vi "Actor Core.vi"(8 "error in":errorcluster, 11 "Elevator Controller in":refnum<class "Sim Display Console Actor.lvclass">) -> (0 "error out":errorcluster, 3 "Actor out":refnum<class "Actor.lvclass">)   [LabVIEW 2019, in "Sim Display Console Actor.lvlib" / "Sim Display Console Actor.lvclass"]
doc: "(<B>Filename</B>: Actor Framework.lvlib:Actor.lvclass:Actor Core.vi)\n\nReceives messages to the actor, reacts to them, and initiates any error handling that may shut the actor down.\n\nDescendant classes may override this VI to append parallel tasks for the actor to complete while it handles messages. Overrides use the Call Parent Method node."
uses:
  Sim Display Console Actor.lvclass
  <vilib>/ActorFramework/Actor/Actor.lvclass
  <vilib>/ActorFramework/Stop Msg/Stop Msg.lvclass
  Display Console Actor/Display Console Actor/Display Console Actor.lvclass
  C:/Workspace/CLA/Elevator AF 3rd/Display Console Actor/Display Console Actor/Display Console Actor.lvclass
  C:/Program Files (x86)/National Instruments/LabVIEW 2019/vi.lib/ActorFramework/Actor/Actor.lvclass
  Elevator Controller/Elevator Controller Messages/Get Elevator Location Msg/Get Elevator Location Msg.lvclass
  Elevator Controller/Elevator Controller Messages/Set Elevator Position Msg/Set Elevator Position Msg.lvclass
  Floors -Enum.ctl
  Elevator Direction.ctl
panel:
  out "Door Open":bool
  out "Emergency":bool
  out "Elevator Direction":T1
  out "Elevator Location":T2
  out "Timing":dbl
  # "[Covers: UI3]"
  # "[Covers: UI3C]"
  # "[Covers: UI3A] \n[Covers: UI3A1] \n[Covers: UI3A2]"
  # "[Covers: UI3D] \n[Covers: UI3D1]"
  # "[Covers: UI3B]"
  # "[Covers: UI3E]"
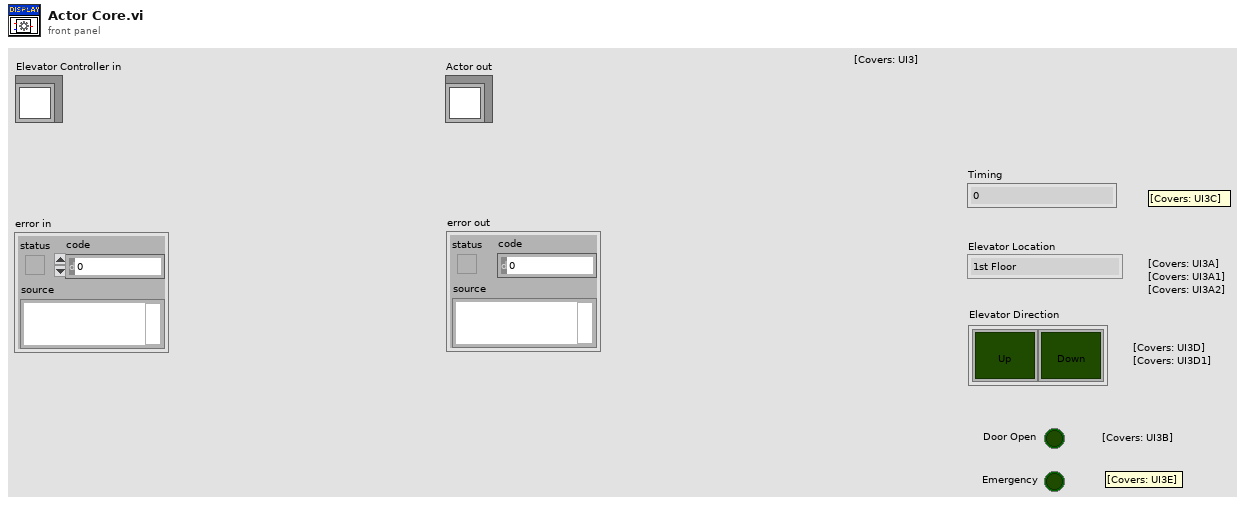
[diagram p1: front panel]
types:
  T1 = typedef "Sim Display Console Actor.lvlib/Sim Display Console Actor.lvclass/Elevator Direction.ctl" = cluster{"Open Door":bool, "Close Door":bool}
  T2 = typedef "Sim Display Console Actor.lvlib/Sim Display Console Actor.lvclass/Floors -Enum.ctl" = enum16{"1st Floor", "2nd Floor", "3rd Floor", "4th Floor"}
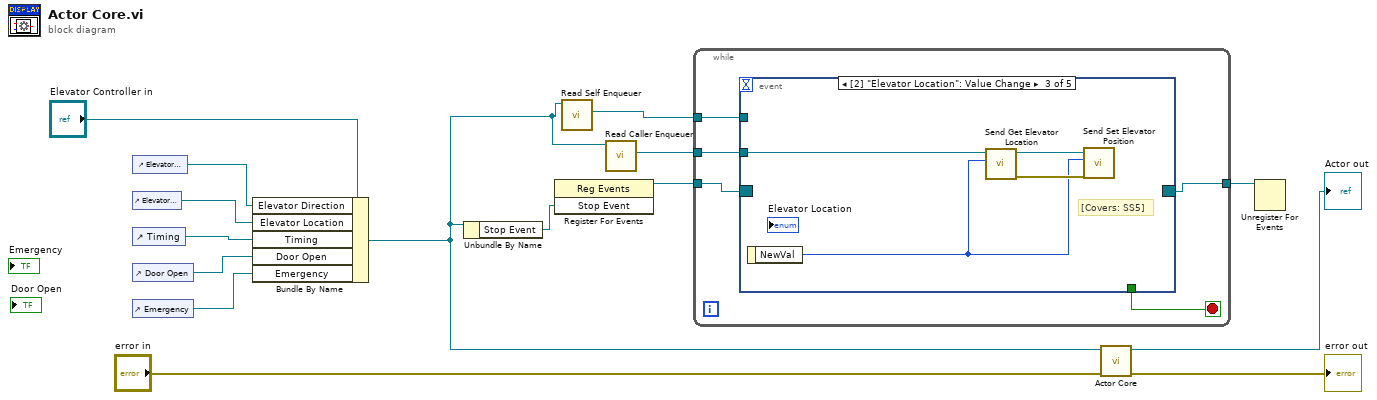
[diagram p0: block diagram]
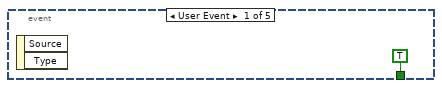
[diagram p2: hidden frame]
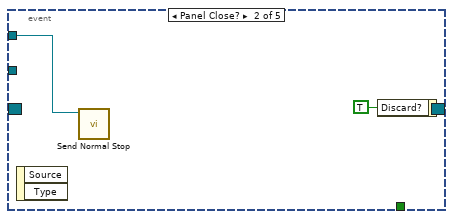
[diagram p3: hidden frame]
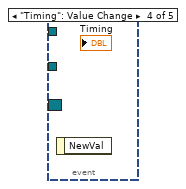
[diagram p4: hidden frame]
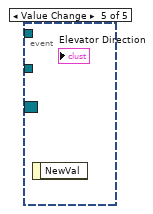
[diagram p5: hidden frame]
diagram:
  n1 = control-ref of="Elevator Direction"() -> (w7:refnum<vi>)
  n2 = control-ref of="Elevator Location"() -> (w6:refnum<vi>)
  n3 = control-ref of="Timing"() -> (w5:refnum<vi>)
  n4 = control-ref of="Door Open"() -> (w4:refnum<vi>)
  n5 = control-ref of="Emergency"() -> (w3:refnum<vi>)
  n6 = Bundle By Name(cluster="Elevator Controller in", "Elevator Direction"=w7, "Elevator Location"=w6, "Timing"=w5, "Door Open"=w4, "Emergency"=w3) -> (w2:refnum<class "Sim Display Console Actor.lvclass">)
  n7 = Unbundle By Name(w2) -> ("Stop Event"=w10:refnum<user-event>)
  n8 = register-events(w10) -> (reference out=w12:refnum<event-registration>)  [unwired: 2 in, 1 out]
  n9 = call <vilib>:"Read Self Enqueuer.vi"("Actor"=w2) -> ("Self Enqueuer"=w9:refnum<class "Message Enqueuer.lvclass">)  [unwired: 10 in]
  n10 = call <vilib>:"Read Caller Enqueuer.vi"("Actor"=w2) -> ("Caller Enqueuer"=w1:refnum<class "Message Enqueuer.lvclass">)  [unwired: 10 in]
  n11 = while {
    tunnel: w12 -> [w20]
    tunnel: [w19] -> w11
    tunnel: w9 -> [w18]
    tunnel: w1 -> [w16]
    stop <- w17 stop-if-true
    n12 = event shown="[2] \"Elevator Location\": Value Change" {
      selector: w20 -> [_ _ _ _ _]
      dyn-events: [_ _ _ _ _] -> w19
      timeout: _ -> [_ _ _ _ _]
      tunnel: w18 -> [_ w22 _ _ _]
      tunnel: [TRUE _ _ _ _] -> w17
      tunnel: w16 -> [_ _ w27 _ _]
      event User Event {
        n13 = event-data() -> ()  [unwired: 1 in, 2 out]
      }
      event Panel Close? {
        n14 = event-data() -> ()  [unwired: 1 in, 2 out]
        n15 = call <vilib>:"Send Normal Stop.vi"("Message Enqueuer"=w22) -> ()  [unwired: 10 in, 1 out]
        n16 = event-data("Discard?"=TRUE) -> ()  [unwired: 1 in, 1 out]
      }
      event Value Change {
        # "[Covers: SS5]"
        n17 = event-data() -> ("NewVal"=w24:T2)  [unwired: 1 in]
        n18 = call "Send Get Elevator Location.vi"("Elevator Location"=w24, "Message Enqueuer"=w27) -> ("error out"=w26:errorcluster, "Message Enqueuer out"=w25:refnum<class "Message Enqueuer.lvclass">)  [unwired: 8 in]
        n19 = call "Send Set Elevator Position.vi"("error in (no error)"=w26, "Elevator Location"=w24, "Message Enqueuer"=w25) -> ()  [unwired: 7 in, 2 out]
      }
      event "Timing": Value Change {
        n20 = event-data() -> ()  [unwired: 1 in, 1 out]
      }
      event Value Change {
        n21 = event-data() -> ()  [unwired: 1 in, 1 out]
      }
    }
  }
  n22 = call-parent "Actor Core.vi"("error in"="error in", "Actor in"=w2) -> ("error out"=→"error out":errorcluster, "Actor out"=→"Actor out":refnum<class "Actor.lvclass">)  [unwired: 8 in]
  n23 = Unregister For Events(event registration refnum=w11) -> ()  [unwired: 1 in, 1 out]
